vi "teste initail 50.vi"() -> ()   [LabVIEW 2026]
uses:
  <vilib>/numeric/Random Number (Range) DBL.vi
  <vilib>/ptbypt/NI_PtbyPt.lvlib
  <vilib>/Analysis/NI_AALBase.lvlib
panel:
  out "Histogram Graph":T1(graph) caption="Graphe de l'histogramme"
  in  "stop":bool
  out "Graphe déroulant":dbl(graph)
  in  "mi cours":bool
  in  "Énum":T2(ring)=enum."sinus"
  in  "piezo start":bool
  in  "frequency sin X":dbl=2.0 caption="fréquence" format="%0.2f"
  in  "delta sin X":dbl=1000.0
  out "dt sin X":dbl=7.597
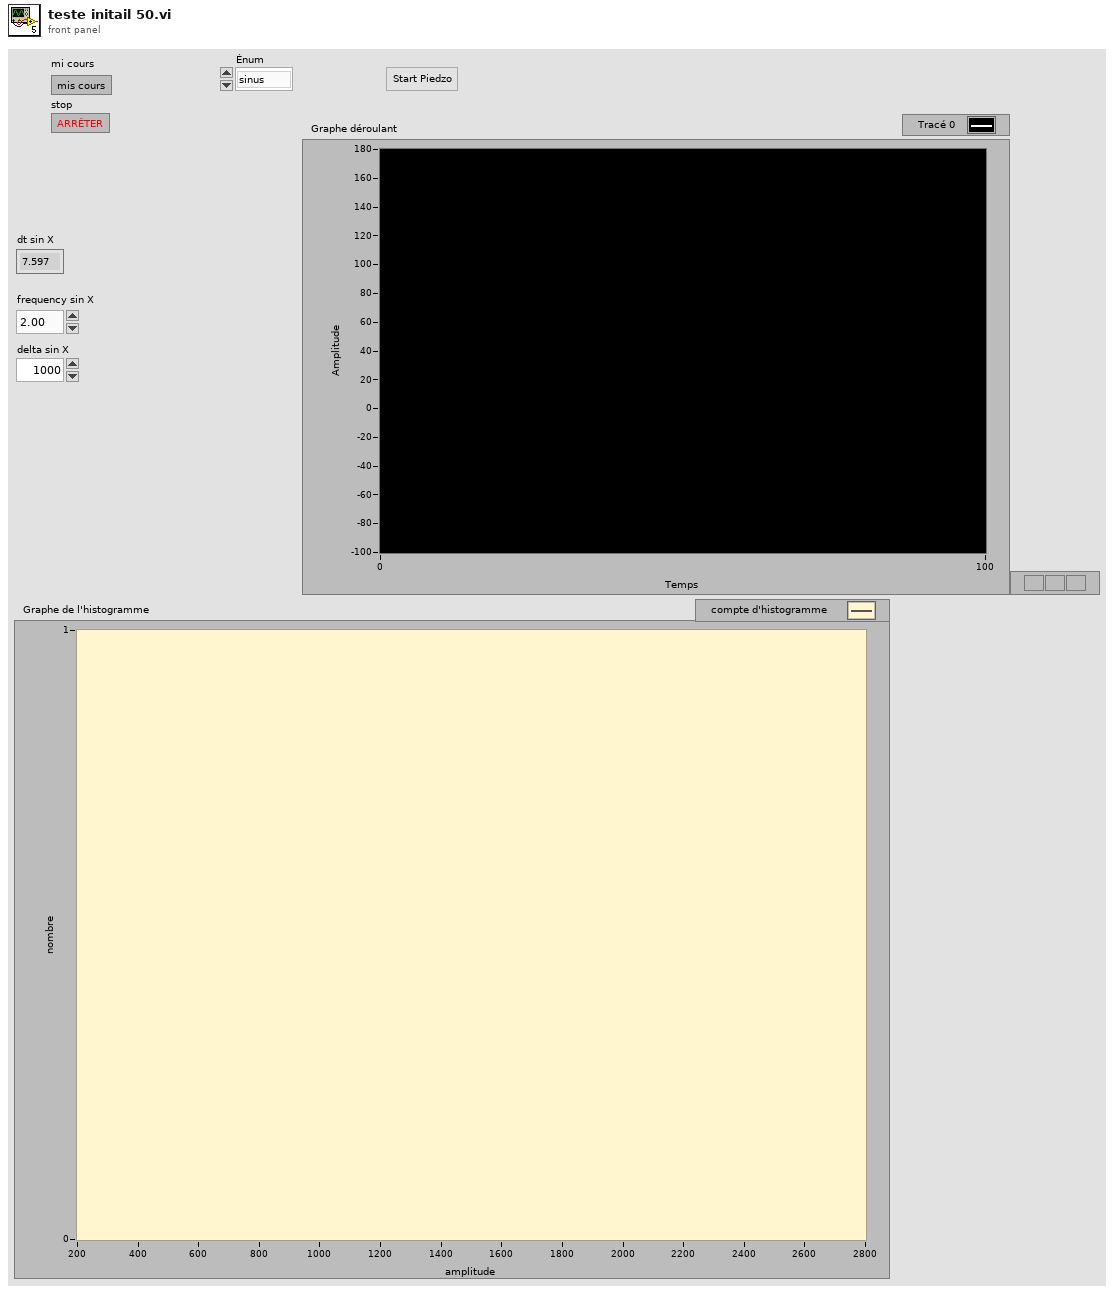
[diagram p1: front panel]
types:
  T1 = cluster{"X Values":dbl[], "Histogram: h(x)":i32[]}
  T2 = enum16{"initial", "aléatoire", "gaussien", "sinus"}
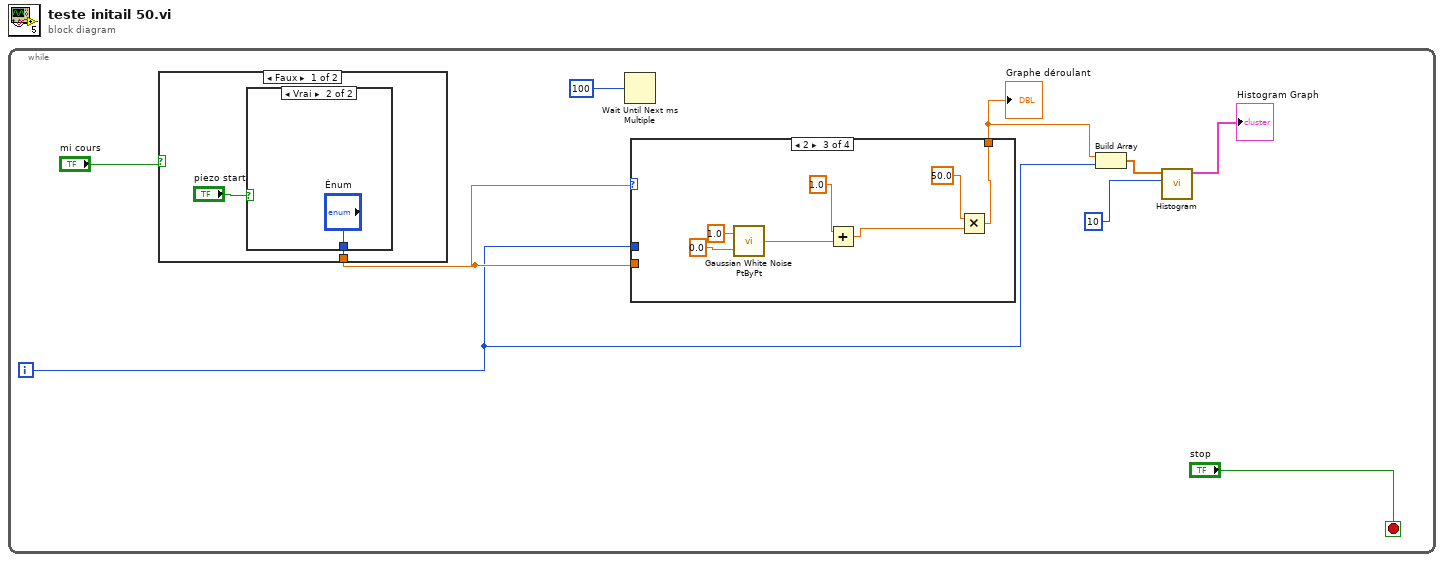
[diagram p0: block diagram]
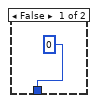
[diagram p2: hidden frame]
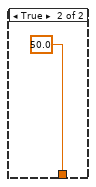
[diagram p3: hidden frame]
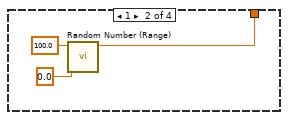
[diagram p5: hidden frame]
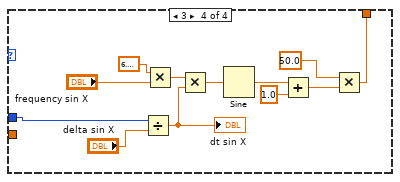
[diagram p6: hidden frame]
diagram:
  n1 = while {
    i -> [w1]
    stop <- "stop" stop-if-true
    n2 = case shown="Faux" "mi cours" {
      tunnel: [w11 50.0] -> w9
      frame False {
        n3 = case shown="Vrai" "piezo start" {
          tunnel: [0 "Énum"] -> w11
          frame False {
          }
          frame True {
          }
        }
      }
      frame True {
      }
    }
    n4 = Wait Until Next ms Multiple(millisecond multiple=u32 100 ("n millisecondes")) -> ()  [unwired: 1 out]
    n5 = case shown="2" w9 {
      tunnel: [w15 w17 w22 w26] -> w3
      tunnel: w1 -> [_ _ _ w27]
      tunnel: w9 -> [w15 _ _ _]
      frame 0, Default {
      }
      frame 1 {
        n6 = call-poly <vilib>:"Random Number (Range).vi"("lower bound (0)"=0.0, "upper bound (100)"=100.0) -> ("number"=w17:dbl)  [unwired: 9 in]
      }
      frame 2 {
        n7 = call <vilib>:"Gaussian White Noise PtByPt.vi"("seed"=0.0, "standard deviation"=1.0) -> ("Gaussian white noise"=w21:dbl)  [unwired: 1 in]
        n8 = Add(x=1.0, y=w21) -> (x+y=w19:dbl)
        n9 = Multiply(x=50.0, y=w19) -> (x*y=w22:dbl)
      }
      frame 3 {
        n10 = Divide(x=w27, y="delta sin X") -> (x/y=w34:dbl)
        "dt sin X" <- w34
        n11 = Multiply(x=6.283185307179586, y="frequency sin X") -> (x*y=w36:dbl)
        n12 = Multiply(x=w36, y=w34) -> (x*y=w33:dbl)
        n13 = Sine(x=w33) -> (sin(x)=w32:dbl)
        n14 = Add(x=w32, y=1.0) -> (x+y=w31:dbl)
        n15 = Multiply(x=50.0, y=w31) -> (x*y=w26:dbl)
      }
    }
    "Graphe déroulant" <- w3
    n16 = Build Array(w3, w1) -> (w2:dbl[])
    n17 = call <vilib>:"Histogram.vi"("intervals"=10, "X"=w2) -> ("Histogram Graph"=→"Histogram Graph":T1)  [unwired: 6 in, 3 out]
  }
